vi "Parlog_creation.vi"(0 "DAC Range Setting":u8(knob)=3 scale=0.0..3.0, 1 "DAC and AD Settings":i32(slide)=3 scale=0.0..3.0, 2 "AD 7730 Bit Settings":i32(slide) scale=0.0..1.0, 3 "predicted time [ms] to finalize DAQ":dbl, 4 "Measured Time for DAQ [ms]":u32, 5 "start time":i64, 6 "single channel voltage factor":dbl=1.0, 7 "Single Channel Voltage Output AO":tag="Dev1/ao0", 8 "single channel number":i64=14, 10 "maximum voltage @ 10MW single channel":dbl=10.0 format="%#_13g", 14 "sample_rate":dbl, 15 "pulse_length":dbl, 16 "sample_period":dbl) -> (9 "chanDescs_defaultInd":T5(array[cluster])=[{"name"="HBCm_U30_01", "active"=1, "physicalQuantity"={"type"="A"}}, {"name"="HBCm_U30_02", "active"=1, "physicalQuantity"={"type"="A"}}, {"name"="HBCm_U30_03", "active"=1, "physicalQuantity"={"type"="A"}}, {"name"="HBCm_U30_04", "active"=1, "physicalQuantity"={"type"="A"}}, {"name"="HBCm_U30_05", "active"=1, "physicalQuantity"={"type"="A"}}, {"name"="HBCm_U30_06", "active"=1, "physicalQuantity"={"type"="A"}}, {"name"="HBCm_U30_07", "active"=1, "physicalQuantity"={"type"="A"}}, {"name"="HBCm_U30_08", "active"=1, "physicalQuantity"={"type"="A"}}, {"name"="HBCm_U30_09", "active"=1, "physicalQuantity"={"type"="A"}}, {"name"="HBCm_U30_10", "active"=1, "physicalQuantity"={"type"="A"}}, {"name"="HBCm_U30_11", "active"=1, "physicalQuantity"={"type"="A"}}, {"name"="HBCm_U30_12", "active"=1, "physicalQuantity"={"type"="A"}}, {"name"="HBCm_U30_13", "active"=1, "physicalQuantity"={"type"="A"}}, {"name"="HBCm_U30_14", "active"=1, "physicalQuantity"={"type"="A"}}, {"name"="HBCm_U30_15", "active"=1, "physicalQuantity"={"type"="A"}}, {"name"="HBCm_U30_16", "active"=1, "physicalQuantity"={"type"="A"}}, {"name"="HBCm_U30_17", "active"=1, "physicalQuantity"={"type"="A"}}, {"name"="HBCm_U30_18", "active"=1, "physicalQuantity"={"type"="A"}}, {"name"="HBCm_U30_19", "active"=1, "physicalQuantity"={"type"="A"}}, {"name"="HBCm_U30_20", "active"=1, "physicalQuantity"={"type"="A"}}, {"name"="HBCm_U30_21", "active"=1, "physicalQuantity"={"type"="A"}}, {"name"="HBCm_U30_22", "active"=1, "physicalQuantity"={"type"="A"}}, {"name"="HBCm_U30_23", "active"=1, "physicalQuantity"={"type"="A"}}, {"name"="HBCm_U30_24", "active"=1, "physicalQuantity"={"type"="A"}}, {"name"="HBCm_U30_25", "active"=1, "physicalQuantity"={"type"="A"}}, {"name"="HBCm_U30_26", "active"=1, "physicalQuantity"={"type"="A"}}, {"name"="HBCm_U30_27", "active"=1, "physicalQuantity"={"type"="A"}}, {"name"="HBCm_U30_28", "active"=1, "physicalQuantity"={"type"="A"}}, {"name"="HBCm_U30_29", "active"=1, "physicalQuantity"={"type"="A"}}, {"name"="HBCm_U30_30", "active"=1, "physicalQuantity"={"type"="A"}}, {"name"="HBCm_U30_31", "active"=1, "physicalQuantity"={"type"="A"}}, {"name"="HBCm_U30_32", "active"=1, "physicalQuantity"={"type"="A"}}, {"name"="VBCm_V21_01", "active"=1, "physicalQuantity"={"type"="A"}}, {"name"="VBCm_V21_02", "active"=1, "physicalQuantity"={"type"="A"}}, {"name"="VBCm_V21_03", "active"=1, "physicalQuantity"={"type"="A"}}, {"name"="VBCm_V21_04", "active"=1, "physicalQuantity"={"type"="A"}}, {"name"="VBCm_V21_05", "active"=1, "physicalQuantity"={"type"="A"}}, {"name"="VBCm_V21_06", "active"=1, "physicalQuantity"={"type"="A"}}, {"name"="VBCm_V21_07", "active"=1, "physicalQuantity"={"type"="A"}}, {"name"="VBCm_V21_08", "active"=1, "physicalQuantity"={"type"="A"}}, {"name"="VBCm_V21_09", "active"=1, "physicalQuantity"={"type"="A"}}, {"name"="VBCm_V21_10", "active"=1, "physicalQuantity"={"type"="A"}}, {"name"="VBCm_V21_11", "active"=1, "physicalQuantity"={"type"="A"}}, {"name"="VBCm_V21_12", "active"=1, "physicalQuantity"={"type"="A"}}, {"name"="VBCm_V21_13", "active"=1, "physicalQuantity"={"type"="A"}}, {"name"="VBCm_V21_14", "active"=1, "physicalQuantity"={"type"="A"}}, {"name"="VBCm_V21_15", "active"=1, "physicalQuantity"={"type"="A"}}, {"name"="VBCm_V21_16", "active"=1, "physicalQuantity"={"type"="A"}}, {"name"="VBCm_V21_17", "active"=1, "physicalQuantity"={"type"="A"}}, {"name"="VBCm_V21_18", "active"=1, "physicalQuantity"={"type"="A"}}, {"name"="VBCm_V21_19", "active"=1, "physicalQuantity"={"type"="A"}}, {"name"="VBCm_V21_20", "active"=1, "physicalQuantity"={"type"="A"}}, {"name"="VBCm_V21_21", "active"=1, "physicalQuantity"={"type"="A"}}, {"name"="VBCm_V21_22", "active"=1, "physicalQuantity"={"type"="A"}}, {"name"="VBCm_V21_23", "active"=1, "physicalQuantity"={"type"="A"}}, {"name"="VBCm_V21_24", "active"=1, "physicalQuantity"={"type"="A"}}, {"name"="VBCm_V21_25", "active"=1, "physicalQuantity"={"type"="A"}}, {"name"="VBCm_V21_26", "active"=1, "physicalQuantity"={"type"="A"}}, {"name"="VBCm_V21_27", "active"=1, "physicalQuantity"={"type"="A"}}, {"name"="VBCm_V21_28", "active"=1, "physicalQuantity"={"type"="A"}}, {"name"="VBCm_V21_29", "active"=1, "physicalQuantity"={"type"="A"}}, {"name"="VBCm_V21_30", "active"=1, "physicalQuantity"={"type"="A"}}, {"name"="VBCm_V21_31", "active"=1, "physicalQuantity"={"type"="A"}}, {"name"="VBCm_V21_32", "active"=1, "physicalQuantity"={"type"="A"}}, {"name"="VBCm_V21_33", "active"=1, "physicalQuantity"={"type"="A"}}, {"name"="VBCm_V21_34", "active"=1, "physicalQuantity"={"type"="A"}}, {"name"="VBCm_V21_35", "active"=1, "physicalQuantity"={"type"="A"}}, {"name"="VBCm_V21_36", "active"=1, "physicalQuantity"={"type"="A"}}, {"name"="VBCm_V21_37", "active"=1, "physicalQuantity"={"type"="A"}}, {"name"="VBCm_V21_38", "active"=1, "physicalQuantity"={"type"="A"}}, {"name"="VBCm_V21_39", "active"=1, "physicalQuantity"={"type"="A"}}, {"name"="VBCm_V21_40", "active"=1, "physicalQuantity"={"type"="A"}}, {"name"="VBCs_V21_01", "active"=1, "physicalQuantity"={"type"="A"}}, {"name"="VBCs_V21_02", "active"=1, "physicalQuantity"={"type"="A"}}, {"name"="VBCs_V21_03", "active"=1, "physicalQuantity"={"type"="A"}}, {"name"="VBCs_V21_04", "active"=1, "physicalQuantity"={"type"="A"}}, {"name"="VBCs_V21_05", "active"=1, "physicalQuantity"={"type"="A"}}, {"name"="VBCs_V21_06", "active"=1, "physicalQuantity"={"type"="A"}}, {"name"="VBCs_V21_07", "active"=1, "physicalQuantity"={"type"="A"}}, {"name"="VBCs_V21_08", "active"=1, "physicalQuantity"={"type"="A"}}, {"name"="HBCs_U30_01", "active"=1, "physicalQuantity"={"type"="A"}}, {"name"="HBCs_U30_02", "active"=1, "physicalQuantity"={"type"="A"}}, {"name"="HBCs_U30_03", "active"=1, "physicalQuantity"={"type"="A"}}, {"name"="HBCs_U30_04", "active"=1, "physicalQuantity"={"type"="A"}}, {"name"="HBCs_U30_05", "active"=1, "physicalQuantity"={"type"="A"}}, {"name"="HBCs_U30_06", "active"=1, "physicalQuantity"={"type"="A"}}, {"name"="HBCs_U30_07", "active"=1, "physicalQuantity"={"type"="A"}}, {"name"="HBCs_U30_08", "active"=1, "physicalQuantity"={"type"="A"}}, {"name"="HBCs_U30_09", "active"=1, "physicalQuantity"={"type"="A"}}, {"name"="HBCs_U30_10", "active"=1, "physicalQuantity"={"type"="A"}}, {"name"="HBCs_U30_11", "active"=1, "physicalQuantity"={"type"="A"}}, {"name"="HBCs_U30_12", "active"=1, "physicalQuantity"={"type"="A"}}, {"name"="HBCs_U30_13", "active"=1, "physicalQuantity"={"type"="A"}}, {"name"="HBCs_U30_14", "active"=1, "physicalQuantity"={"type"="A"}}, {"name"="HBCs_U30_15", "active"=1, "physicalQuantity"={"type"="A"}}, {"name"="HBCs_U30_16", "active"=1, "physicalQuantity"={"type"="A"}}, {"name"="Test96", "active"=1, "physicalQuantity"={"type"="A"}}, {"name"="Test97", "active"=0, "physicalQuantity"={"type"=""}}], 11 "chanDescs_ArrayOfArray":T6(array[cluster])=[{"chanDescs"=[{"name"="E_Chan_1", "active"=1}, {"name"="E_Chan_2", "active"=1}, {"name"="E_Chan_3", "active"=1}, {"name"="E_Chan_4", "active"=1}, {"name"="E_Chan_5", "active"=1}, {"name"="E_Chan_6", "active"=1}, {"name"="E_Chan_7", "active"=1}, {"name"="E_Chan_8", "active"=1}, {"name"="E_Chan_9", "active"=1}, {"name"="E_Chan_10", "active"=1}, {"name"="E_Chan_11", "active"=1}, {"name"="E_Chan_12", "active"=1}, {"name"="E_Chan_13", "active"=1}, {"name"="E_Chan_14", "active"=1}, {"name"="E_Chan_15", "active"=1}, {"name"="E_Chan_16", "active"=1}, {"name"="E_Chan_17", "active"=1}, {"name"="E_Chan_18", "active"=1}, {"name"="E_Chan_19", "active"=1}, {"name"="E_Chan_20", "active"=1}, {"name"="E_Chan_21", "active"=1}, {"name"="E_Chan_22", "active"=1}, {"name"="E_Chan_23", "active"=1}, {"name"="E_Chan_24", "active"=1}, {"name"="E_Chan_25", "active"=1}, {"name"="E_Chan_26", "active"=1}, {"name"="E_Chan_27", "active"=1}, {"name"="E_Chan_28", "active"=1}, {"name"="E_Chan_29", "active"=1}, {"name"="E_Chan_30", "active"=1}, {"name"="E_Chan_31", "active"=1}, {"name"="E_Chan_32", "active"=1}, {"name"="E_Chan_33", "active"=1}, {"name"="E_Chan_34", "active"=1}, {"name"="E_Chan_35", "active"=1}, {"name"="E_Chan_36", "active"=1}, {"name"="E_Chan_37", "active"=1}, {"name"="E_Chan_38", "active"=1}, {"name"="E_Chan_39", "active"=1}, {"name"="E_Chan_40", "active"=1}, {"name"="E_Chan_41", "active"=1}, {"name"="E_Chan_42", "active"=1}, {"name"="E_Chan_43", "active"=1}, {"name"="E_Chan_44", "active"=1}, {"name"="E_Chan_45", "active"=1}, {"name"="E_Chan_46", "active"=1}, {"name"="E_Chan_47", "active"=1}, {"name"="E_Chan_48", "active"=1}, {"name"="E_Chan_49", "active"=1}, {"name"="E_Chan_50", "active"=1}, {"name"="E_Chan_51", "active"=1}, {"name"="E_Chan_52", "active"=1}, {"name"="E_Chan_53", "active"=1}, {"name"="E_Chan_54", "active"=1}, {"name"="E_Chan_55", "active"=1}, {"name"="E_Chan_56", "active"=1}, {"name"="E_Chan_57", "active"=1}, {"name"="E_Chan_58", "active"=1}, {"name"="E_Chan_59", "active"=1}, {"name"="E_Chan_60", "active"=1}, {"name"="E_Chan_61", "active"=1}, {"name"="E_Chan_62", "active"=1}, {"name"="E_Chan_63", "active"=1}, {"name"="E_Chan_64", "active"=1}, {"name"="E_Chan_65", "active"=1}, {"name"="E_Chan_66", "active"=1}, {"name"="E_Chan_67", "active"=1}, {"name"="E_Chan_68", "active"=1}, {"name"="E_Chan_69", "active"=1}, {"name"="E_Chan_70", "active"=1}, {"name"="E_Chan_71", "active"=1}, {"name"="E_Chan_72", "active"=1}, {"name"="E_Chan_73", "active"=1}, {"name"="E_Chan_74", "active"=1}, {"name"="E_Chan_75", "active"=1}, {"name"="E_Chan_76", "active"=1}, {"name"="E_Chan_77", "active"=1}, {"name"="E_Chan_78", "active"=1}, {"name"="E_Chan_79", "active"=1}, {"name"="E_Chan_80", "active"=1}, {"name"="E_Chan_81", "active"=1}, {"name"="E_Chan_82", "active"=1}, {"name"="E_Chan_83", "active"=1}, {"name"="E_Chan_84", "active"=1}, {"name"="E_Chan_85", "active"=1}, {"name"="E_Chan_86", "active"=1}, {"name"="E_Chan_87", "active"=1}, {"name"="E_Chan_88", "active"=1}, {"name"="E_Chan_89", "active"=1}, {"name"="E_Chan_90", "active"=1}, {"name"="E_Chan_91", "active"=1}, {"name"="E_Chan_92", "active"=1}, {"name"="E_Chan_93", "active"=1}, {"name"="E_Chan_94", "active"=1}, {"name"="E_Chan_95", "active"=1}, {"name"="E_Chan_96", "active"=1}, {"name"="E_Chan_97", "active"=1}, {"name"="E_Chan_98", "active"=1}, {"name"="E_Chan_99", "active"=1}, {"name"="E_Chan_100", "active"=1}, {"name"="E_Chan_101", "active"=1}, {"name"="E_Chan_102", "active"=1}, {"name"="E_Chan_103", "active"=1}, {"name"="E_Chan_104", "active"=1}, {"name"="E_Chan_105", "active"=1}, {"name"="E_Chan_106", "active"=1}, {"name"="E_Chan_107", "active"=1}, {"name"="E_Chan_108", "active"=1}, {"name"="E_Chan_109", "active"=1}, {"name"="E_Chan_110", "active"=1}, {"name"="E_Chan_111", "active"=1}, {"name"="E_Chan_112", "active"=1}, {"name"="E_Chan_113", "active"=1}, {"name"="E_Chan_114", "active"=1}, {"name"="E_Chan_115", "active"=1}, {"name"="E_Chan_116", "active"=1}, {"name"="E_Chan_117", "active"=1}, {"name"="E_Chan_118", "active"=1}, {"name"="E_Chan_119", "active"=1}, {"name"="E_Chan_120", "active"=1}, {"name"="E_Chan_121", "active"=1}, {"name"="E_Chan_122", "active"=1}, {"name"="E_Chan_123", "active"=1}, {"name"="E_Chan_124", "active"=1}, {"name"="E_Chan_125", "active"=1}, {"name"="E_Chan_126", "active"=1}, {"name"="E_Chan_127", "active"=1}, {"name"="E_Chan_128", "active"=1}]}], 12 "cluster":T1, 13 "reduced cluster array":T3(array[cluster]), 17 "reduced cluster":T4, 18 "chanDescsInd":T5(array[cluster])=[{"name"="HBCm_U30_01", "active"=1, "physicalQuantity"={"type"="A"}}, {"name"="HBCm_U30_02", "active"=1, "physicalQuantity"={"type"="A"}}, {"name"="HBCm_U30_03", "active"=1, "physicalQuantity"={"type"="A"}}, {"name"="HBCm_U30_04", "active"=1, "physicalQuantity"={"type"="A"}}, {"name"="HBCm_U30_05", "active"=1, "physicalQuantity"={"type"="A"}}, {"name"="HBCm_U30_06", "active"=1, "physicalQuantity"={"type"="A"}}, {"name"="HBCm_U30_07", "active"=1, "physicalQuantity"={"type"="A"}}, {"name"="HBCm_U30_08", "active"=1, "physicalQuantity"={"type"="A"}}, {"name"="HBCm_U30_09", "active"=1, "physicalQuantity"={"type"="A"}}, {"name"="HBCm_U30_10", "active"=1, "physicalQuantity"={"type"="A"}}, {"name"="HBCm_U30_11", "active"=1, "physicalQuantity"={"type"="A"}}, {"name"="HBCm_U30_12", "active"=1, "physicalQuantity"={"type"="A"}}, {"name"="HBCm_U30_013", "active"=1, "physicalQuantity"={"type"="A"}}, {"name"="HBCm_U30_14", "active"=1, "physicalQuantity"={"type"="A"}}, {"name"="HBCm_U30_15", "active"=1, "physicalQuantity"={"type"="A"}}, {"name"="HBCm_U30_16", "active"=1, "physicalQuantity"={"type"="A"}}, {"name"="HBCm_U30_17", "active"=1, "physicalQuantity"={"type"="A"}}, {"name"="HBCm_U30_18", "active"=1, "physicalQuantity"={"type"="A"}}, {"name"="HBCm_U30_19", "active"=1, "physicalQuantity"={"type"="A"}}, {"name"="HBCm_U30_20", "active"=1, "physicalQuantity"={"type"="A"}}, {"name"="HBCm_U30_21", "active"=1, "physicalQuantity"={"type"="A"}}, {"name"="HBCm_U30_22", "active"=1, "physicalQuantity"={"type"="A"}}, {"name"="HBCm_U30_23", "active"=1, "physicalQuantity"={"type"="A"}}, {"name"="HBCm_U30_24", "active"=1, "physicalQuantity"={"type"="A"}}, {"name"="HBCm_U30_25", "active"=1, "physicalQuantity"={"type"="A"}}, {"name"="HBCm_U30_26", "active"=1, "physicalQuantity"={"type"="A"}}, {"name"="HBCm_U30_27", "active"=1, "physicalQuantity"={"type"="A"}}, {"name"="HBCm_U30_28", "active"=1, "physicalQuantity"={"type"="A"}}, {"name"="HBCm_U30_29", "active"=1, "physicalQuantity"={"type"="A"}}, {"name"="HBCm_U30_30", "active"=1, "physicalQuantity"={"type"="A"}}, {"name"="HBCm_U30_31", "active"=1, "physicalQuantity"={"type"="A"}}, {"name"="HBCm_U30_32", "active"=1, "physicalQuantity"={"type"="A"}}, {"name"="VBCm_V21_01", "active"=1, "physicalQuantity"={"type"="A"}}, {"name"="VBCm_V21_02", "active"=1, "physicalQuantity"={"type"="A"}}, {"name"="VBCm_V21_03", "active"=1, "physicalQuantity"={"type"="A"}}, {"name"="VBCm_V21_04", "active"=1, "physicalQuantity"={"type"="A"}}, {"name"="VBCm_V21_05", "active"=1, "physicalQuantity"={"type"="A"}}, {"name"="VBCm_V21_06", "active"=1, "physicalQuantity"={"type"="A"}}, {"name"="VBCm_V21_07", "active"=1, "physicalQuantity"={"type"="A"}}, {"name"="VBCm_V21_08", "active"=1, "physicalQuantity"={"type"="A"}}, {"name"="VBCm_V21_09", "active"=1, "physicalQuantity"={"type"="A"}}, {"name"="VBCm_V21_10", "active"=1, "physicalQuantity"={"type"="A"}}, {"name"="VBCm_V21_11", "active"=1, "physicalQuantity"={"type"="A"}}, {"name"="VBCm_V21_12", "active"=1, "physicalQuantity"={"type"="A"}}, {"name"="VBCm_V21_13", "active"=1, "physicalQuantity"={"type"="A"}}, {"name"="VBCm_V21_14", "active"=1, "physicalQuantity"={"type"="A"}}, {"name"="VBCm_V21_15", "active"=1, "physicalQuantity"={"type"="A"}}, {"name"="VBCm_V21_16", "active"=1, "physicalQuantity"={"type"="A"}}, {"name"="VBCm_V21_17", "active"=1, "physicalQuantity"={"type"="A"}}, {"name"="VBCm_V21_18", "active"=1, "physicalQuantity"={"type"="A"}}, {"name"="VBCm_V21_19", "active"=1, "physicalQuantity"={"type"="A"}}, {"name"="VBCm_V21_20", "active"=1, "physicalQuantity"={"type"="A"}}, {"name"="VBCm_V21_21", "active"=1, "physicalQuantity"={"type"="A"}}, {"name"="VBCm_V21_22", "active"=1, "physicalQuantity"={"type"="A"}}, {"name"="VBCm_V21_23", "active"=1, "physicalQuantity"={"type"="A"}}, {"name"="VBCm_V21_24", "active"=1, "physicalQuantity"={"type"="A"}}, {"name"="VBCm_V21_25", "active"=1, "physicalQuantity"={"type"="A"}}, {"name"="VBCm_V21_26", "active"=1, "physicalQuantity"={"type"="A"}}, {"name"="VBCm_V21_27", "active"=1, "physicalQuantity"={"type"="A"}}, {"name"="VBCm_V21_28", "active"=1, "physicalQuantity"={"type"="A"}}, {"name"="VBCm_V21_29", "active"=1, "physicalQuantity"={"type"="A"}}, {"name"="VBCm_V21_30", "active"=1, "physicalQuantity"={"type"="A"}}, {"name"="VBCm_V21_31", "active"=1, "physicalQuantity"={"type"="A"}}, {"name"="VBCm_V21_32", "active"=1, "physicalQuantity"={"type"="A"}}, {"name"="VBCm_V21_33", "active"=1, "physicalQuantity"={"type"="A"}}, {"name"="VBCm_V21_34", "active"=1, "physicalQuantity"={"type"="A"}}, {"name"="VBCm_V21_35", "active"=1, "physicalQuantity"={"type"="A"}}, {"name"="VBCm_V21_36", "active"=1, "physicalQuantity"={"type"="A"}}, {"name"="VBCm_V21_37", "active"=1, "physicalQuantity"={"type"="A"}}, {"name"="VBCm_V21_38", "active"=1, "physicalQuantity"={"type"="A"}}, {"name"="VBCm_V21_39", "active"=1, "physicalQuantity"={"type"="A"}}, {"name"="VBCm_V21_40", "active"=1, "physicalQuantity"={"type"="A"}}, {"name"="VBCs_V21_01", "active"=1, "physicalQuantity"={"type"="A"}}, {"name"="VBCs_V21_02", "active"=1, "physicalQuantity"={"type"="A"}}, {"name"="VBCs_V21_03", "active"=1, "physicalQuantity"={"type"="A"}}, {"name"="VBCs_V21_04", "active"=1, "physicalQuantity"={"type"="A"}}, {"name"="VBCs_V21_05", "active"=1, "physicalQuantity"={"type"="A"}}, {"name"="VBCs_V21_06", "active"=1, "physicalQuantity"={"type"="A"}}, {"name"="VBCs_V21_07", "active"=1, "physicalQuantity"={"type"="A"}}, {"name"="VBCs_V21_08", "active"=1, "physicalQuantity"={"type"="A"}}, {"name"="HBCs_U30_01", "active"=1, "physicalQuantity"={"type"="A"}}, {"name"="HBCs_U30_02", "active"=1, "physicalQuantity"={"type"="A"}}, {"name"="HBCs_U30_03", "active"=1, "physicalQuantity"={"type"="A"}}, {"name"="HBCs_U30_04", "active"=1, "physicalQuantity"={"type"="A"}}, {"name"="HBCs_U30_05", "active"=1, "physicalQuantity"={"type"="A"}}, {"name"="HBCs_U30_06", "active"=1, "physicalQuantity"={"type"="A"}}, {"name"="HBCs_U30_07", "active"=1, "physicalQuantity"={"type"="A"}}, {"name"="HBCs_U30_08", "active"=1, "physicalQuantity"={"type"="A"}}, {"name"="HBCs_U30_09", "active"=1, "physicalQuantity"={"type"="A"}}, {"name"="HBCs_U30_10", "active"=1, "physicalQuantity"={"type"="A"}}, {"name"="HBCs_U30_11", "active"=1, "physicalQuantity"={"type"="A"}}, {"name"="HBCs_U30_12", "active"=1, "physicalQuantity"={"type"="A"}}, {"name"="HBCs_U30_13", "active"=1, "physicalQuantity"={"type"="A"}}, {"name"="HBCs_U30_14", "active"=1, "physicalQuantity"={"type"="A"}}, {"name"="HBCs_U30_15", "active"=1, "physicalQuantity"={"type"="A"}}, {"name"="HBCs_U30_16", "active"=1, "physicalQuantity"={"type"="A"}}], 19 "cluster array":T2(array[cluster]))   [LabVIEW 2014]
panel:
  out "cluster json":string
  out "cluster array json":string
  out "chanDescs 2":cluster{"name":string, "active":i32}[](array[cluster])=[{"name"="E_Chan_1", "active"=1}, {"name"="E_Chan_2", "active"=1}, {"name"="E_Chan_3", "active"=1}, {"name"="E_Chan_4", "active"=1}, {"name"="E_Chan_5", "active"=1}, {"name"="E_Chan_6", "active"=1}, {"name"="E_Chan_7", "active"=1}, {"name"="E_Chan_8", "active"=1}, {"name"="E_Chan_9", "active"=1}, {"name"="E_Chan_10", "active"=1}, {"name"="E_Chan_11", "active"=1}, {"name"="E_Chan_12", "active"=1}, {"name"="E_Chan_13", "active"=1}, {"name"="E_Chan_14", "active"=1}, {"name"="E_Chan_15", "active"=1}, {"name"="E_Chan_16", "active"=1}, {"name"="E_Chan_17", "active"=1}, {"name"="E_Chan_18", "active"=1}, {"name"="E_Chan_19", "active"=1}, {"name"="E_Chan_20", "active"=1}, {"name"="E_Chan_21", "active"=1}, {"name"="E_Chan_22", "active"=1}, {"name"="E_Chan_23", "active"=1}, {"name"="E_Chan_24", "active"=1}, {"name"="E_Chan_25", "active"=1}, {"name"="E_Chan_26", "active"=1}, {"name"="E_Chan_27", "active"=1}, {"name"="E_Chan_28", "active"=1}, {"name"="E_Chan_29", "active"=1}, {"name"="E_Chan_30", "active"=1}, {"name"="E_Chan_31", "active"=1}, {"name"="E_Chan_32", "active"=1}, {"name"="E_Chan_33", "active"=1}, {"name"="E_Chan_34", "active"=1}, {"name"="E_Chan_35", "active"=1}, {"name"="E_Chan_36", "active"=1}, {"name"="E_Chan_37", "active"=1}, {"name"="E_Chan_38", "active"=1}, {"name"="E_Chan_39", "active"=1}, {"name"="E_Chan_40", "active"=1}, {"name"="E_Chan_41", "active"=1}, {"name"="E_Chan_42", "active"=1}, {"name"="E_Chan_43", "active"=1}, {"name"="E_Chan_44", "active"=1}, {"name"="E_Chan_45", "active"=1}, {"name"="E_Chan_46", "active"=1}, {"name"="E_Chan_47", "active"=1}, {"name"="E_Chan_48", "active"=1}, {"name"="E_Chan_49", "active"=1}, {"name"="E_Chan_50", "active"=1}, {"name"="E_Chan_51", "active"=1}, {"name"="E_Chan_52", "active"=1}, {"name"="E_Chan_53", "active"=1}, {"name"="E_Chan_54", "active"=1}, {"name"="E_Chan_55", "active"=1}, {"name"="E_Chan_56", "active"=1}, {"name"="E_Chan_57", "active"=1}, {"name"="E_Chan_58", "active"=1}, {"name"="E_Chan_59", "active"=1}, {"name"="E_Chan_60", "active"=1}, {"name"="E_Chan_61", "active"=1}, {"name"="E_Chan_62", "active"=1}, {"name"="E_Chan_63", "active"=1}, {"name"="E_Chan_64", "active"=1}, {"name"="E_Chan_65", "active"=1}, {"name"="E_Chan_66", "active"=1}, {"name"="E_Chan_67", "active"=1}, {"name"="E_Chan_68", "active"=1}, {"name"="E_Chan_69", "active"=1}, {"name"="E_Chan_70", "active"=1}, {"name"="E_Chan_71", "active"=1}, {"name"="E_Chan_72", "active"=1}, {"name"="E_Chan_73", "active"=1}, {"name"="E_Chan_74", "active"=1}, {"name"="E_Chan_75", "active"=1}, {"name"="E_Chan_76", "active"=1}, {"name"="E_Chan_77", "active"=1}, {"name"="E_Chan_78", "active"=1}, {"name"="E_Chan_79", "active"=1}, {"name"="E_Chan_80", "active"=1}, {"name"="E_Chan_81", "active"=1}, {"name"="E_Chan_82", "active"=1}, {"name"="E_Chan_83", "active"=1}, {"name"="E_Chan_84", "active"=1}, {"name"="E_Chan_85", "active"=1}, {"name"="E_Chan_86", "active"=1}, {"name"="E_Chan_87", "active"=1}, {"name"="E_Chan_88", "active"=1}, {"name"="E_Chan_89", "active"=1}, {"name"="E_Chan_90", "active"=1}, {"name"="E_Chan_91", "active"=1}, {"name"="E_Chan_92", "active"=1}, {"name"="E_Chan_93", "active"=1}, {"name"="E_Chan_94", "active"=1}, {"name"="E_Chan_95", "active"=1}, {"name"="E_Chan_96", "active"=1}, {"name"="E_Chan_97", "active"=1}, {"name"="E_Chan_98", "active"=1}, {"name"="E_Chan_99", "active"=1}, {"name"="E_Chan_100", "active"=1}, {"name"="E_Chan_101", "active"=1}, {"name"="E_Chan_102", "active"=1}, {"name"="E_Chan_103", "active"=1}, {"name"="E_Chan_104", "active"=1}, {"name"="E_Chan_105", "active"=1}, {"name"="E_Chan_106", "active"=1}, {"name"="E_Chan_107", "active"=1}, {"name"="E_Chan_108", "active"=1}, {"name"="E_Chan_109", "active"=1}, {"name"="E_Chan_110", "active"=1}, {"name"="E_Chan_111", "active"=1}, {"name"="E_Chan_112", "active"=1}, {"name"="E_Chan_113", "active"=1}, {"name"="E_Chan_114", "active"=1}, {"name"="E_Chan_115", "active"=1}, {"name"="E_Chan_116", "active"=1}, {"name"="E_Chan_117", "active"=1}, {"name"="E_Chan_118", "active"=1}, {"name"="E_Chan_119", "active"=1}, {"name"="E_Chan_120", "active"=1}, {"name"="E_Chan_121", "active"=1}, {"name"="E_Chan_122", "active"=1}, {"name"="E_Chan_123", "active"=1}, {"name"="E_Chan_124", "active"=1}, {"name"="E_Chan_125", "active"=1}, {"name"="E_Chan_126", "active"=1}, {"name"="E_Chan_127", "active"=1}, {"name"="E_Chan_128", "active"=1}]
  in  "chanDescs":T5(array[cluster])=[{"name"="HBCm_U30_01", "active"=1, "physicalQuantity"={"type"="A"}}, {"name"="HBCm_U30_02", "active"=1, "physicalQuantity"={"type"="A"}}, {"name"="HBCm_U30_03", "active"=1, "physicalQuantity"={"type"="A"}}, {"name"="HBCm_U30_04", "active"=1, "physicalQuantity"={"type"="A"}}, {"name"="HBCm_U30_05", "active"=1, "physicalQuantity"={"type"="A"}}, {"name"="HBCm_U30_06", "active"=1, "physicalQuantity"={"type"="A"}}, {"name"="HBCm_U30_07", "active"=1, "physicalQuantity"={"type"="A"}}, {"name"="HBCm_U30_08", "active"=1, "physicalQuantity"={"type"="A"}}, {"name"="HBCm_U30_09", "active"=1, "physicalQuantity"={"type"="A"}}, {"name"="HBCm_U30_10", "active"=1, "physicalQuantity"={"type"="A"}}, {"name"="HBCm_U30_11", "active"=1, "physicalQuantity"={"type"="A"}}, {"name"="HBCm_U30_12", "active"=1, "physicalQuantity"={"type"="A"}}, {"name"="HBCm_U30_013", "active"=1, "physicalQuantity"={"type"="A"}}, {"name"="HBCm_U30_14", "active"=1, "physicalQuantity"={"type"="A"}}, {"name"="HBCm_U30_15", "active"=1, "physicalQuantity"={"type"="A"}}, {"name"="HBCm_U30_16", "active"=1, "physicalQuantity"={"type"="A"}}, {"name"="HBCm_U30_17", "active"=1, "physicalQuantity"={"type"="A"}}, {"name"="HBCm_U30_18", "active"=1, "physicalQuantity"={"type"="A"}}, {"name"="HBCm_U30_19", "active"=1, "physicalQuantity"={"type"="A"}}, {"name"="HBCm_U30_20", "active"=1, "physicalQuantity"={"type"="A"}}, {"name"="HBCm_U30_21", "active"=1, "physicalQuantity"={"type"="A"}}, {"name"="HBCm_U30_22", "active"=1, "physicalQuantity"={"type"="A"}}, {"name"="HBCm_U30_23", "active"=1, "physicalQuantity"={"type"="A"}}, {"name"="HBCm_U30_24", "active"=1, "physicalQuantity"={"type"="A"}}, {"name"="HBCm_U30_25", "active"=1, "physicalQuantity"={"type"="A"}}, {"name"="HBCm_U30_26", "active"=1, "physicalQuantity"={"type"="A"}}, {"name"="HBCm_U30_27", "active"=1, "physicalQuantity"={"type"="A"}}, {"name"="HBCm_U30_28", "active"=1, "physicalQuantity"={"type"="A"}}, {"name"="HBCm_U30_29", "active"=1, "physicalQuantity"={"type"="A"}}, {"name"="HBCm_U30_30", "active"=1, "physicalQuantity"={"type"="A"}}, {"name"="HBCm_U30_31", "active"=1, "physicalQuantity"={"type"="A"}}, {"name"="HBCm_U30_32", "active"=1, "physicalQuantity"={"type"="A"}}, {"name"="VBCm_V21_01", "active"=1, "physicalQuantity"={"type"="A"}}, {"name"="VBCm_V21_02", "active"=1, "physicalQuantity"={"type"="A"}}, {"name"="VBCm_V21_03", "active"=1, "physicalQuantity"={"type"="A"}}, {"name"="VBCm_V21_04", "active"=1, "physicalQuantity"={"type"="A"}}, {"name"="VBCm_V21_05", "active"=1, "physicalQuantity"={"type"="A"}}, {"name"="VBCm_V21_06", "active"=1, "physicalQuantity"={"type"="A"}}, {"name"="VBCm_V21_07", "active"=1, "physicalQuantity"={"type"="A"}}, {"name"="VBCm_V21_08", "active"=1, "physicalQuantity"={"type"="A"}}, {"name"="VBCm_V21_09", "active"=1, "physicalQuantity"={"type"="A"}}, {"name"="VBCm_V21_10", "active"=1, "physicalQuantity"={"type"="A"}}, {"name"="VBCm_V21_11", "active"=1, "physicalQuantity"={"type"="A"}}, {"name"="VBCm_V21_12", "active"=1, "physicalQuantity"={"type"="A"}}, {"name"="VBCm_V21_13", "active"=1, "physicalQuantity"={"type"="A"}}, {"name"="VBCm_V21_14", "active"=1, "physicalQuantity"={"type"="A"}}, {"name"="VBCm_V21_15", "active"=1, "physicalQuantity"={"type"="A"}}, {"name"="VBCm_V21_16", "active"=1, "physicalQuantity"={"type"="A"}}, {"name"="VBCm_V21_17", "active"=1, "physicalQuantity"={"type"="A"}}, {"name"="VBCm_V21_18", "active"=1, "physicalQuantity"={"type"="A"}}, {"name"="VBCm_V21_19", "active"=1, "physicalQuantity"={"type"="A"}}, {"name"="VBCm_V21_20", "active"=1, "physicalQuantity"={"type"="A"}}, {"name"="VBCm_V21_21", "active"=1, "physicalQuantity"={"type"="A"}}, {"name"="VBCm_V21_22", "active"=1, "physicalQuantity"={"type"="A"}}, {"name"="VBCm_V21_23", "active"=1, "physicalQuantity"={"type"="A"}}, {"name"="VBCm_V21_24", "active"=1, "physicalQuantity"={"type"="A"}}, {"name"="VBCm_V21_25", "active"=1, "physicalQuantity"={"type"="A"}}, {"name"="VBCm_V21_26", "active"=1, "physicalQuantity"={"type"="A"}}, {"name"="VBCm_V21_27", "active"=1, "physicalQuantity"={"type"="A"}}, {"name"="VBCm_V21_28", "active"=1, "physicalQuantity"={"type"="A"}}, {"name"="VBCm_V21_29", "active"=1, "physicalQuantity"={"type"="A"}}, {"name"="VBCm_V21_30", "active"=1, "physicalQuantity"={"type"="A"}}, {"name"="VBCm_V21_31", "active"=1, "physicalQuantity"={"type"="A"}}, {"name"="VBCm_V21_32", "active"=1, "physicalQuantity"={"type"="A"}}, {"name"="VBCm_V21_33", "active"=1, "physicalQuantity"={"type"="A"}}, {"name"="VBCm_V21_34", "active"=1, "physicalQuantity"={"type"="A"}}, {"name"="VBCm_V21_35", "active"=1, "physicalQuantity"={"type"="A"}}, {"name"="VBCm_V21_36", "active"=1, "physicalQuantity"={"type"="A"}}, {"name"="VBCm_V21_37", "active"=1, "physicalQuantity"={"type"="A"}}, {"name"="VBCm_V21_38", "active"=1, "physicalQuantity"={"type"="A"}}, {"name"="VBCm_V21_39", "active"=1, "physicalQuantity"={"type"="A"}}, {"name"="VBCm_V21_40", "active"=1, "physicalQuantity"={"type"="A"}}, {"name"="VBCs_V21_01", "active"=1, "physicalQuantity"={"type"="A"}}, {"name"="VBCs_V21_02", "active"=1, "physicalQuantity"={"type"="A"}}, {"name"="VBCs_V21_03", "active"=1, "physicalQuantity"={"type"="A"}}, {"name"="VBCs_V21_04", "active"=1, "physicalQuantity"={"type"="A"}}, {"name"="VBCs_V21_05", "active"=1, "physicalQuantity"={"type"="A"}}, {"name"="VBCs_V21_06", "active"=1, "physicalQuantity"={"type"="A"}}, {"name"="VBCs_V21_07", "active"=1, "physicalQuantity"={"type"="A"}}, {"name"="VBCs_V21_08", "active"=1, "physicalQuantity"={"type"="A"}}, {"name"="HBCs_U30_01", "active"=1, "physicalQuantity"={"type"="A"}}, {"name"="HBCs_U30_02", "active"=1, "physicalQuantity"={"type"="A"}}, {"name"="HBCs_U30_03", "active"=1, "physicalQuantity"={"type"="A"}}, {"name"="HBCs_U30_04", "active"=1, "physicalQuantity"={"type"="A"}}, {"name"="HBCs_U30_05", "active"=1, "physicalQuantity"={"type"="A"}}, {"name"="HBCs_U30_06", "active"=1, "physicalQuantity"={"type"="A"}}, {"name"="HBCs_U30_07", "active"=1, "physicalQuantity"={"type"="A"}}, {"name"="HBCs_U30_08", "active"=1, "physicalQuantity"={"type"="A"}}, {"name"="HBCs_U30_09", "active"=1, "physicalQuantity"={"type"="A"}}, {"name"="HBCs_U30_10", "active"=1, "physicalQuantity"={"type"="A"}}, {"name"="HBCs_U30_11", "active"=1, "physicalQuantity"={"type"="A"}}, {"name"="HBCs_U30_12", "active"=1, "physicalQuantity"={"type"="A"}}, {"name"="HBCs_U30_13", "active"=1, "physicalQuantity"={"type"="A"}}, {"name"="HBCs_U30_14", "active"=1, "physicalQuantity"={"type"="A"}}, {"name"="HBCs_U30_15", "active"=1, "physicalQuantity"={"type"="A"}}, {"name"="HBCs_U30_16", "active"=1, "physicalQuantity"={"type"="A"}}]
  in  "Pre-start time (ms) of DAQ Typically set to 1000 ms":i32=5000
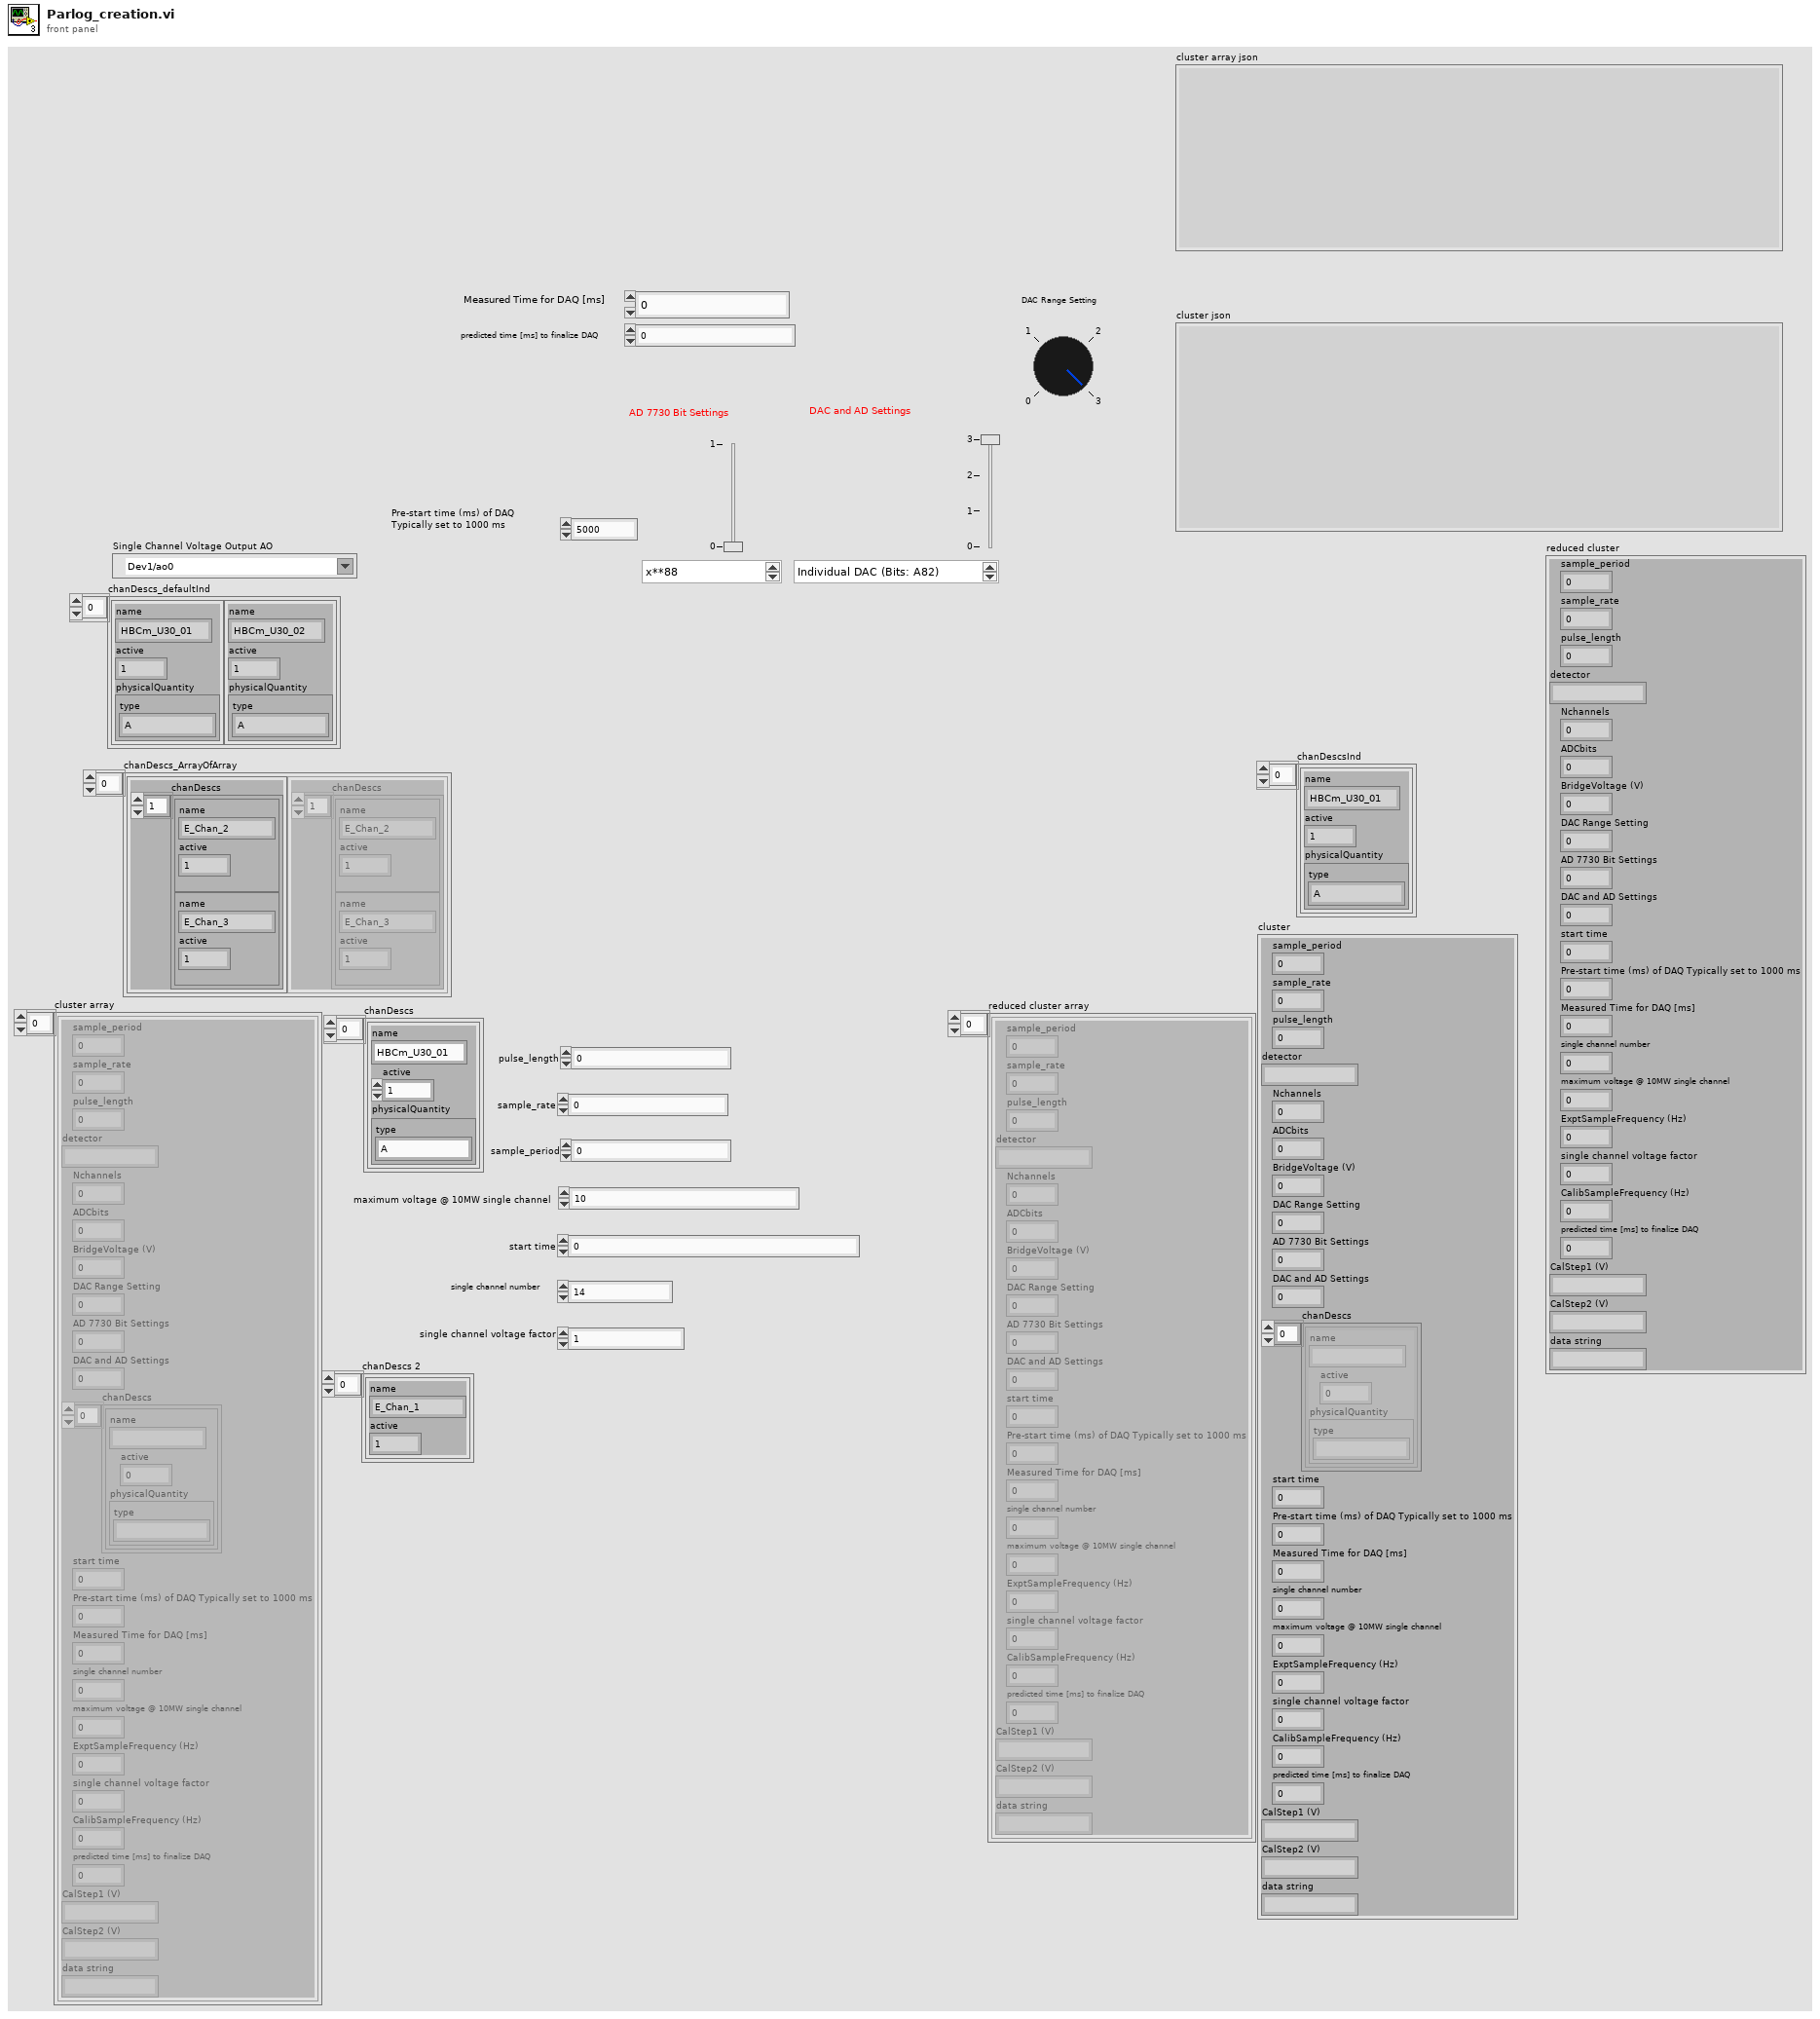
[diagram p1: front panel]
types:
  T1 = cluster{"sample_period":dbl, "sample_rate":dbl, "pulse_length":dbl, "detector":string, "Nchannels":i16, "ADCbits":i16, "BridgeVoltage (V)":sgl, "DAC Range Setting":u8, "AD 7730 Bit Settings":i32, "DAC and AD Settings":i32, "chanDescs":cluster{"name":string, "active":i32, "physicalQuantity":cluster{"type":string}}[], "start time":i64, "Pre-start time (ms) of DAQ Typically set to 1000 ms":i32, "Measured Time for DAQ [ms] ":u32, "single channel number":i64, "maximum voltage @ 10MW single channel":dbl, "ExptSampleFrequency (Hz)":sgl, "single channel voltage factor":dbl, "CalibSampleFrequency (Hz)":sgl, "predicted time [ms] to finalize DAQ":dbl, "CalStep1 (V)":string, "CalStep2 (V)":string, "data string":string}
  T2 = cluster{"sample_period":dbl, "sample_rate":dbl, "pulse_length":dbl, "detector":string, "Nchannels":i16, "ADCbits":i16, "BridgeVoltage (V)":sgl, "DAC Range Setting":u8, "AD 7730 Bit Settings":i32, "DAC and AD Settings":i32, "chanDescs":cluster{"name":string, "active":i32, "physicalQuantity":cluster{"type":string}}[], "start time":i64, "Pre-start time (ms) of DAQ Typically set to 1000 ms":i32, "Measured Time for DAQ [ms] ":u32, "single channel number":i64, "maximum voltage @ 10MW single channel":dbl, "ExptSampleFrequency (Hz)":sgl, "single channel voltage factor":dbl, "CalibSampleFrequency (Hz)":sgl, "predicted time [ms] to finalize DAQ":dbl, "CalStep1 (V)":string, "CalStep2 (V)":string, "data string":string}[]
  T3 = cluster{"sample_period":dbl, "sample_rate":dbl, "pulse_length":dbl, "detector":string, "Nchannels":i16, "ADCbits":i16, "BridgeVoltage (V)":sgl, "DAC Range Setting":u8, "AD 7730 Bit Settings":i32, "DAC and AD Settings":i32, "start time":i64, "Pre-start time (ms) of DAQ Typically set to 1000 ms":i32, "Measured Time for DAQ [ms] ":u32, "single channel number":i64, "maximum voltage @ 10MW single channel":dbl, "ExptSampleFrequency (Hz)":sgl, "single channel voltage factor":dbl, "CalibSampleFrequency (Hz)":sgl, "predicted time [ms] to finalize DAQ":dbl, "CalStep1 (V)":string, "CalStep2 (V)":string, "data string":string}[]
  T4 = cluster{"sample_period":dbl, "sample_rate":dbl, "pulse_length":dbl, "detector":string, "Nchannels":i16, "ADCbits":i16, "BridgeVoltage (V)":sgl, "DAC Range Setting":u8, "AD 7730 Bit Settings":i32, "DAC and AD Settings":i32, "start time":i64, "Pre-start time (ms) of DAQ Typically set to 1000 ms":i32, "Measured Time for DAQ [ms] ":u32, "single channel number":i64, "maximum voltage @ 10MW single channel":dbl, "ExptSampleFrequency (Hz)":sgl, "single channel voltage factor":dbl, "CalibSampleFrequency (Hz)":sgl, "predicted time [ms] to finalize DAQ":dbl, "CalStep1 (V)":string, "CalStep2 (V)":string, "data string":string}
  T5 = cluster{"name":string, "active":i32, "physicalQuantity":cluster{"type":string}}[]
  T6 = cluster{"chanDescs":cluster{"name":string, "active":i32}[]}[]
  T7 = cluster{"sample_period":dbl, "sample_rate":dbl, "pulse_length":dbl, "detector":string, "NChannels":i16, "ADCBits":i16, "BridgeVoltage (V)":sgl, "DAC Range Setting":u8, "AD 7730 Bit Settings":i32, "DAC and AD Settings":i32, "chanDescs":cluster{"name":string, "active":i32, "physicalQuantity":cluster{"type":string}}[], "start time":i64, "Pre-start time (ms) of DAQ Typically set to 1000 ms":i32, "Measured Time for DAQ [ms] ":u32, "single channel number":i64, "maximum voltage @ 10MW single channel":dbl, "ExptSampleFrequency (Hz)":sgl, "single channel voltage factor":dbl, "CalibSampleFrequency (Hz)":sgl, "predicted time [ms] to finalize DAQ":dbl, "CalStep1 (V)":string, "CalStep2 (V)":string, "data string":string}
  T8 = cluster{"sample_period":dbl, "sample_rate":dbl, "pulse_length":dbl, "detector":string, "NChannels":i16, "ADCBits":i16, "BridgeVoltage (V)":sgl, "DAC Range Setting":u8, "AD 7730 Bit Settings":i32, "DAC and AD Settings":i32, "start time":i64, "Pre-start time (ms) of DAQ Typically set to 1000 ms":i32, "Measured Time for DAQ [ms] ":u32, "single channel number":i64, "maximum voltage @ 10MW single channel":dbl, "ExptSampleFrequency (Hz)":sgl, "single channel voltage factor":dbl, "CalibSampleFrequency (Hz)":sgl, "predicted time [ms] to finalize DAQ":dbl, "CalStep1 (V)":string, "CalStep2 (V)":string, "data string":string}
  T9 = cluster{"sample_period":dbl, "sample_rate":dbl, "pulse_length":dbl, "detector":string, "NChannels":i16, "ADCBits":i16, "BridgeVoltage (V)":sgl, "DAC Range Setting":u8, "AD 7730 Bit Settings":i32, "DAC and AD Settings":i32, "start time":i64, "Pre-start time (ms) of DAQ Typically set to 1000 ms":i32, "Measured Time for DAQ [ms] ":u32, "single channel number":i64, "maximum voltage @ 10MW single channel":dbl, "ExptSampleFrequency (Hz)":sgl, "single channel voltage factor":dbl, "CalibSampleFrequency (Hz)":sgl, "predicted time [ms] to finalize DAQ":dbl, "CalStep1 (V)":string, "CalStep2 (V)":string, "data string":string}[]
  T10 = cluster{"sample_period":dbl, "sample_rate":dbl, "pulse_length":dbl, "detector":string, "NChannels":i16, "ADCBits":i16, "BridgeVoltage (V)":sgl, "DAC Range Setting":u8, "AD 7730 Bit Settings":i32, "DAC and AD Settings":i32, "chanDescs":cluster{"name":string, "active":i32, "physicalQuantity":cluster{"type":string}}[], "start time":i64, "Pre-start time (ms) of DAQ Typically set to 1000 ms":i32, "Measured Time for DAQ [ms] ":u32, "single channel number":i64, "maximum voltage @ 10MW single channel":dbl, "ExptSampleFrequency (Hz)":sgl, "single channel voltage factor":dbl, "CalibSampleFrequency (Hz)":sgl, "predicted time [ms] to finalize DAQ":dbl, "CalStep1 (V)":string, "CalStep2 (V)":string, "data string":string}[]
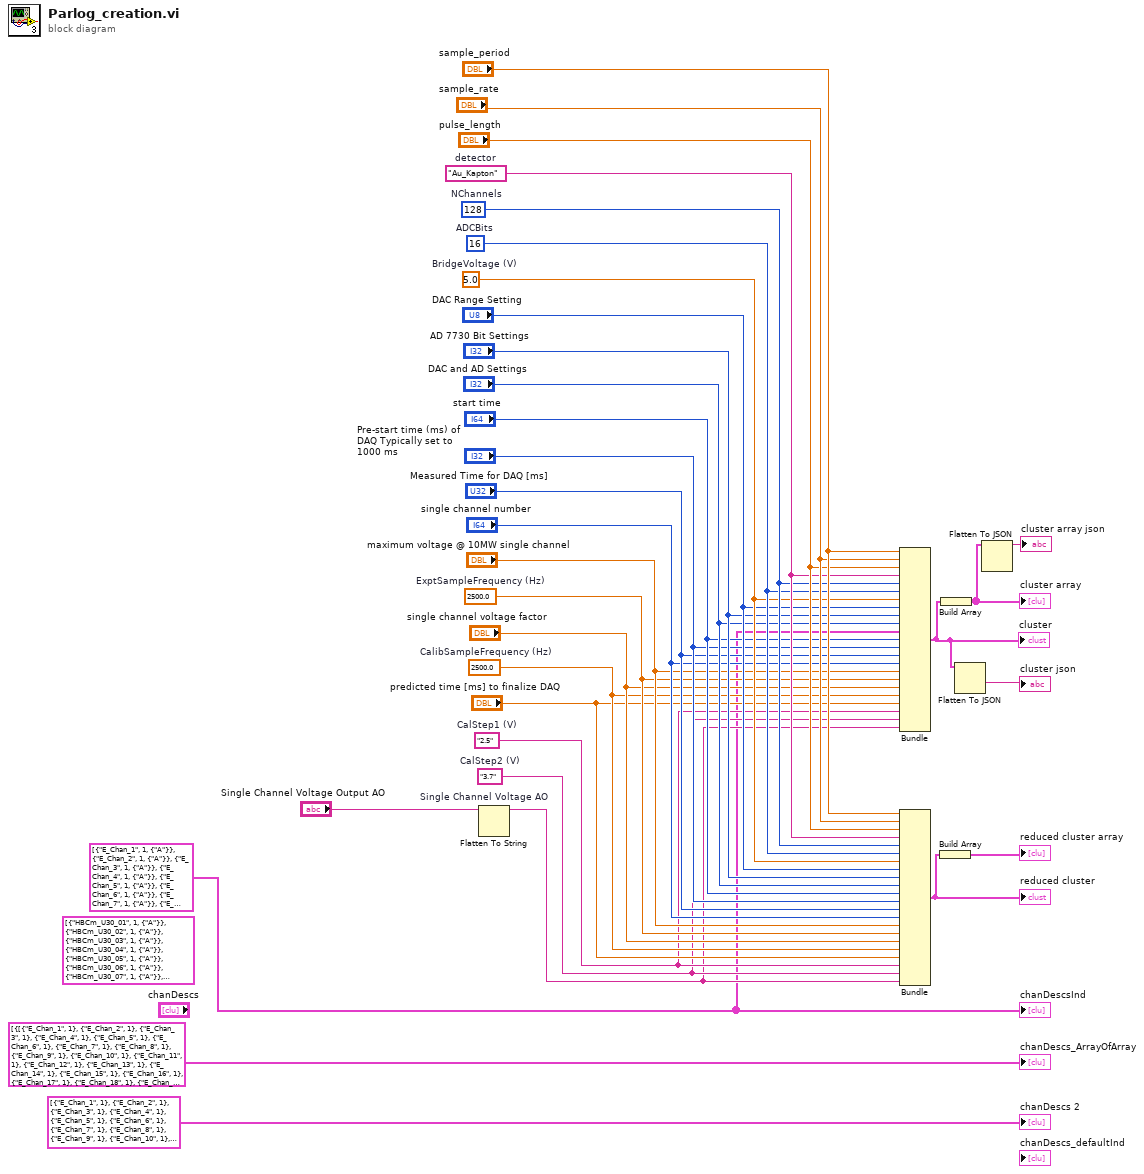
[diagram p0: block diagram]
diagram:
  w1 = T5 [{"name"="E_Chan_1", "active"=1, "physicalQuantity"={"type"="A"}}, {"name"="E_Chan_2", "active"=1, "physicalQuantity"={"type"="A"}}, {"name"="E_Chan_3", "active"=1, "physicalQuantity"={"type"="A"}}, {"name"="E_Chan_4", "active"=1, "physicalQuantity"={"type"="A"}}, {"name"="E_Chan_5", "active"=1, "physicalQuantity"={"type"="A"}}, {"name"="E_Chan_6", "active"=1, "physicalQuantity"={"type"="A"}}, {"name"="E_Chan_7", "active"=1, "physicalQuantity"={"type"="A"}}, {"name"="E_Chan_8", "active"=1, "physicalQuantity"={"type"="A"}}, {"name"="E_Chan_9", "active"=1, "physicalQuantity"={"type"="A"}}, {"name"="E_Chan_10", "active"=1, "physicalQuantity"={"type"="A"}}, {"name"="E_Chan_11", "active"=1, "physicalQuantity"={"type"="A"}}, {"name"="E_Chan_12", "active"=1, "physicalQuantity"={"type"="A"}}, {"name"="E_Chan_13", "active"=1, "physicalQuantity"={"type"="A"}}, {"name"="E_Chan_14", "active"=1, "physicalQuantity"={"type"="A"}}, {"name"="E_Chan_15", "active"=1, "physicalQuantity"={"type"="A"}}, {"name"="E_Chan_16", "active"=1, "physicalQuantity"={"type"="A"}}, {"name"="E_Chan_17", "active"=1, "physicalQuantity"={"type"="A"}}, {"name"="E_Chan_18", "active"=1, "physicalQuantity"={"type"="A"}}, {"name"="E_Chan_19", "active"=1, "physicalQuantity"={"type"="A"}}, {"name"="E_Chan_20", "active"=1, "physicalQuantity"={"type"="A"}}, {"name"="E_Chan_21", "active"=1, "physicalQuantity"={"type"="A"}}, {"name"="E_Chan_22", "active"=1, "physicalQuantity"={"type"="A"}}, {"name"="E_Chan_23", "active"=1, "physicalQuantity"={"type"="A"}}, {"name"="E_Chan_24", "active"=1, "physicalQuantity"={"type"="A"}}, {"name"="E_Chan_25", "active"=1, "physicalQuantity"={"type"="A"}}, {"name"="E_Chan_26", "active"=1, "physicalQuantity"={"type"="A"}}, {"name"="E_Chan_27", "active"=1, "physicalQuantity"={"type"="A"}}, {"name"="E_Chan_28", "active"=1, "physicalQuantity"={"type"="A"}}, {"name"="E_Chan_29", "active"=1, "physicalQuantity"={"type"="A"}}, {"name"="E_Chan_30", "active"=1, "physicalQuantity"={"type"="A"}}, {"name"="E_Chan_31", "active"=1, "physicalQuantity"={"type"="A"}}, {"name"="E_Chan_32", "active"=1, "physicalQuantity"={"type"="A"}}, {"name"="E_Chan_33", "active"=1, "physicalQuantity"={"type"="A"}}, {"name"="E_Chan_34", "active"=1, "physicalQuantity"={"type"="A"}}, {"name"="E_Chan_35", "active"=1, "physicalQuantity"={"type"="A"}}, {"name"="E_Chan_36", "active"=1, "physicalQuantity"={"type"="A"}}, {"name"="E_Chan_37", "active"=1, "physicalQuantity"={"type"="A"}}, {"name"="E_Chan_38", "active"=1, "physicalQuantity"={"type"="A"}}, {"name"="E_Chan_39", "active"=1, "physicalQuantity"={"type"="A"}}, {"name"="E_Chan_40", "active"=1, "physicalQuantity"={"type"="A"}}, {"name"="E_Chan_41", "active"=1, "physicalQuantity"={"type"="A"}}, {"name"="E_Chan_42", "active"=1, "physicalQuantity"={"type"="A"}}, {"name"="E_Chan_43", "active"=1, "physicalQuantity"={"type"="A"}}, {"name"="E_Chan_44", "active"=1, "physicalQuantity"={"type"="A"}}, {"name"="E_Chan_45", "active"=1, "physicalQuantity"={"type"="A"}}, {"name"="E_Chan_46", "active"=1, "physicalQuantity"={"type"="A"}}, {"name"="E_Chan_47", "active"=1, "physicalQuantity"={"type"="A"}}, {"name"="E_Chan_48", "active"=1, "physicalQuantity"={"type"="A"}}, {"name"="E_Chan_49", "active"=1, "physicalQuantity"={"type"="A"}}, {"name"="E_Chan_50", "active"=1, "physicalQuantity"={"type"="A"}}, {"name"="E_Chan_51", "active"=1, "physicalQuantity"={"type"="A"}}, {"name"="E_Chan_52", "active"=1, "physicalQuantity"={"type"="A"}}, {"name"="E_Chan_53", "active"=1, "physicalQuantity"={"type"="A"}}, {"name"="E_Chan_54", "active"=1, "physicalQuantity"={"type"="A"}}, {"name"="E_Chan_55", "active"=1, "physicalQuantity"={"type"="A"}}, {"name"="E_Chan_56", "active"=1, "physicalQuantity"={"type"="A"}}, {"name"="E_Chan_57", "active"=1, "physicalQuantity"={"type"="A"}}, {"name"="E_Chan_58", "active"=1, "physicalQuantity"={"type"="A"}}, {"name"="E_Chan_59", "active"=1, "physicalQuantity"={"type"="A"}}, {"name"="E_Chan_60", "active"=1, "physicalQuantity"={"type"="A"}}, {"name"="E_Chan_61", "active"=1, "physicalQuantity"={"type"="A"}}, {"name"="E_Chan_62", "active"=1, "physicalQuantity"={"type"="A"}}, {"name"="E_Chan_63", "active"=1, "physicalQuantity"={"type"="A"}}, {"name"="E_Chan_64", "active"=1, "physicalQuantity"={"type"="A"}}, {"name"="E_Chan_65", "active"=1, "physicalQuantity"={"type"="A"}}, {"name"="E_Chan_66", "active"=1, "physicalQuantity"={"type"="A"}}, {"name"="E_Chan_67", "active"=1, "physicalQuantity"={"type"="A"}}, {"name"="E_Chan_68", "active"=1, "physicalQuantity"={"type"="A"}}, {"name"="E_Chan_69", "active"=1, "physicalQuantity"={"type"="A"}}, {"name"="E_Chan_70", "active"=1, "physicalQuantity"={"type"="A"}}, {"name"="E_Chan_71", "active"=1, "physicalQuantity"={"type"="A"}}, {"name"="E_Chan_72", "active"=1, "physicalQuantity"={"type"="A"}}, {"name"="E_Chan_73", "active"=1, "physicalQuantity"={"type"="A"}}, {"name"="E_Chan_74", "active"=1, "physicalQuantity"={"type"="A"}}, {"name"="E_Chan_75", "active"=1, "physicalQuantity"={"type"="A"}}, {"name"="E_Chan_76", "active"=1, "physicalQuantity"={"type"="A"}}, {"name"="E_Chan_77", "active"=1, "physicalQuantity"={"type"="A"}}, {"name"="E_Chan_78", "active"=1, "physicalQuantity"={"type"="A"}}, {"name"="E_Chan_79", "active"=1, "physicalQuantity"={"type"="A"}}, {"name"="E_Chan_80", "active"=1, "physicalQuantity"={"type"="A"}}, {"name"="E_Chan_81", "active"=1, "physicalQuantity"={"type"="A"}}, {"name"="E_Chan_82", "active"=1, "physicalQuantity"={"type"="A"}}, {"name"="E_Chan_83", "active"=1, "physicalQuantity"={"type"="A"}}, {"name"="E_Chan_84", "active"=1, "physicalQuantity"={"type"="A"}}, {"name"="E_Chan_85", "active"=1, "physicalQuantity"={"type"="A"}}, {"name"="E_Chan_86", "active"=1, "physicalQuantity"={"type"="A"}}, {"name"="E_Chan_87", "active"=1, "physicalQuantity"={"type"="A"}}, {"name"="E_Chan_88", "active"=1, "physicalQuantity"={"type"="A"}}, {"name"="E_Chan_89", "active"=1, "physicalQuantity"={"type"="A"}}, {"name"="E_Chan_90", "active"=1, "physicalQuantity"={"type"="A"}}, {"name"="E_Chan_91", "active"=1, "physicalQuantity"={"type"="A"}}, {"name"="E_Chan_92", "active"=1, "physicalQuantity"={"type"="A"}}, {"name"="E_Chan_93", "active"=1, "physicalQuantity"={"type"="A"}}, {"name"="E_Chan_94", "active"=1, "physicalQuantity"={"type"="A"}}, {"name"="E_Chan_95", "active"=1, "physicalQuantity"={"type"="A"}}, {"name"="E_Chan_96", "active"=1, "physicalQuantity"={"type"="A"}}, {"name"="E_Chan_97", "active"=1, "physicalQuantity"={"type"="A"}}, {"name"="E_Chan_98", "active"=1, "physicalQuantity"={"type"="A"}}, {"name"="E_Chan_99", "active"=1, "physicalQuantity"={"type"="A"}}, {"name"="E_Chan_100", "active"=1, "physicalQuantity"={"type"="A"}}, {"name"="E_Chan_101", "active"=1, "physicalQuantity"={"type"="A"}}, {"name"="E_Chan_102", "active"=1, "physicalQuantity"={"type"="A"}}, {"name"="E_Chan_103", "active"=1, "physicalQuantity"={"type"="A"}}, {"name"="E_Chan_104", "active"=1, "physicalQuantity"={"type"="A"}}, {"name"="E_Chan_105", "active"=1, "physicalQuantity"={"type"="A"}}, {"name"="E_Chan_106", "active"=1, "physicalQuantity"={"type"="A"}}, {"name"="E_Chan_107", "active"=1, "physicalQuantity"={"type"="A"}}, {"name"="E_Chan_108", "active"=1, "physicalQuantity"={"type"="A"}}, {"name"="E_Chan_109", "active"=1, "physicalQuantity"={"type"="A"}}, {"name"="E_Chan_110", "active"=1, "physicalQuantity"={"type"="A"}}, {"name"="E_Chan_111", "active"=1, "physicalQuantity"={"type"="A"}}, {"name"="E_Chan_112", "active"=1, "physicalQuantity"={"type"="A"}}, {"name"="E_Chan_113", "active"=1, "physicalQuantity"={"type"="A"}}, {"name"="E_Chan_114", "active"=1, "physicalQuantity"={"type"="A"}}, {"name"="E_Chan_115", "active"=1, "physicalQuantity"={"type"="A"}}, {"name"="E_Chan_116", "active"=1, "physicalQuantity"={"type"="A"}}, {"name"="E_Chan_117", "active"=1, "physicalQuantity"={"type"="A"}}, {"name"="E_Chan_118", "active"=1, "physicalQuantity"={"type"="A"}}, {"name"="E_Chan_119", "active"=1, "physicalQuantity"={"type"="A"}}, {"name"="E_Chan_120", "active"=1, "physicalQuantity"={"type"="A"}}, {"name"="E_Chan_121", "active"=1, "physicalQuantity"={"type"="A"}}, {"name"="E_Chan_122", "active"=1, "physicalQuantity"={"type"="A"}}, {"name"="E_Chan_123", "active"=1, "physicalQuantity"={"type"="A"}}, {"name"="E_Chan_124", "active"=1, "physicalQuantity"={"type"="A"}}, {"name"="E_Chan_125", "active"=1, "physicalQuantity"={"type"="A"}}, {"name"="E_Chan_126", "active"=1, "physicalQuantity"={"type"="A"}}, {"name"="E_Chan_127", "active"=1, "physicalQuantity"={"type"="A"}}, {"name"="E_Chan_128", "active"=1, "physicalQuantity"={"type"="A"}}] ("chanDescs")
  (unwired) T5 [{"name"="HBCm_U30_01", "active"=1, "physicalQuantity"={"type"="A"}}, {"name"="HBCm_U30_02", "active"=1, "physicalQuantity"={"type"="A"}}, {"name"="HBCm_U30_03", "active"=1, "physicalQuantity"={"type"="A"}}, {"name"="HBCm_U30_04", "active"=1, "physicalQuantity"={"type"="A"}}, {"name"="HBCm_U30_05", "active"=1, "physicalQuantity"={"type"="A"}}, {"name"="HBCm_U30_06", "active"=1, "physicalQuantity"={"type"="A"}}, {"name"="HBCm_U30_07", "active"=1, "physicalQuantity"={"type"="A"}}, {"name"="HBCm_U30_08", "active"=1, "physicalQuantity"={"type"="A"}}, {"name"="HBCm_U30_09", "active"=1, "physicalQuantity"={"type"="A"}}, {"name"="HBCm_U30_10", "active"=1, "physicalQuantity"={"type"="A"}}, {"name"="HBCm_U30_11", "active"=1, "physicalQuantity"={"type"="A"}}, {"name"="HBCm_U30_12", "active"=1, "physicalQuantity"={"type"="A"}}, {"name"="HBCm_U30_013", "active"=1, "physicalQuantity"={"type"="A"}}, {"name"="HBCm_U30_14", "active"=1, "physicalQuantity"={"type"="A"}}, {"name"="HBCm_U30_15", "active"=1, "physicalQuantity"={"type"="A"}}, {"name"="HBCm_U30_16", "active"=1, "physicalQuantity"={"type"="A"}}, {"name"="HBCm_U30_17", "active"=1, "physicalQuantity"={"type"="A"}}, {"name"="HBCm_U30_18", "active"=1, "physicalQuantity"={"type"="A"}}, {"name"="HBCm_U30_19", "active"=1, "physicalQuantity"={"type"="A"}}, {"name"="HBCm_U30_20", "active"=1, "physicalQuantity"={"type"="A"}}, {"name"="HBCm_U30_21", "active"=1, "physicalQuantity"={"type"="A"}}, {"name"="HBCm_U30_22", "active"=1, "physicalQuantity"={"type"="A"}}, {"name"="HBCm_U30_23", "active"=1, "physicalQuantity"={"type"="A"}}, {"name"="HBCm_U30_24", "active"=1, "physicalQuantity"={"type"="A"}}, {"name"="HBCm_U30_25", "active"=1, "physicalQuantity"={"type"="A"}}, {"name"="HBCm_U30_26", "active"=1, "physicalQuantity"={"type"="A"}}, {"name"="HBCm_U30_27", "active"=1, "physicalQuantity"={"type"="A"}}, {"name"="HBCm_U30_28", "active"=1, "physicalQuantity"={"type"="A"}}, {"name"="HBCm_U30_29", "active"=1, "physicalQuantity"={"type"="A"}}, {"name"="HBCm_U30_30", "active"=1, "physicalQuantity"={"type"="A"}}, {"name"="HBCm_U30_31", "active"=1, "physicalQuantity"={"type"="A"}}, {"name"="HBCm_U30_32", "active"=1, "physicalQuantity"={"type"="A"}}, {"name"="VBCm_V21_01", "active"=1, "physicalQuantity"={"type"="A"}}, {"name"="VBCm_V21_02", "active"=1, "physicalQuantity"={"type"="A"}}, {"name"="VBCm_V21_03", "active"=1, "physicalQuantity"={"type"="A"}}, {"name"="VBCm_V21_04", "active"=1, "physicalQuantity"={"type"="A"}}, {"name"="VBCm_V21_05", "active"=1, "physicalQuantity"={"type"="A"}}, {"name"="VBCm_V21_06", "active"=1, "physicalQuantity"={"type"="A"}}, {"name"="VBCm_V21_07", "active"=1, "physicalQuantity"={"type"="A"}}, {"name"="VBCm_V21_08", "active"=1, "physicalQuantity"={"type"="A"}}, {"name"="VBCm_V21_09", "active"=1, "physicalQuantity"={"type"="A"}}, {"name"="VBCm_V21_10", "active"=1, "physicalQuantity"={"type"="A"}}, {"name"="VBCm_V21_11", "active"=1, "physicalQuantity"={"type"="A"}}, {"name"="VBCm_V21_12", "active"=1, "physicalQuantity"={"type"="A"}}, {"name"="VBCm_V21_13", "active"=1, "physicalQuantity"={"type"="A"}}, {"name"="VBCm_V21_14", "active"=1, "physicalQuantity"={"type"="A"}}, {"name"="VBCm_V21_15", "active"=1, "physicalQuantity"={"type"="A"}}, {"name"="VBCm_V21_16", "active"=1, "physicalQuantity"={"type"="A"}}, {"name"="VBCm_V21_17", "active"=1, "physicalQuantity"={"type"="A"}}, {"name"="VBCm_V21_18", "active"=1, "physicalQuantity"={"type"="A"}}, {"name"="VBCm_V21_19", "active"=1, "physicalQuantity"={"type"="A"}}, {"name"="VBCm_V21_20", "active"=1, "physicalQuantity"={"type"="A"}}, {"name"="VBCm_V21_21", "active"=1, "physicalQuantity"={"type"="A"}}, {"name"="VBCm_V21_22", "active"=1, "physicalQuantity"={"type"="A"}}, {"name"="VBCm_V21_23", "active"=1, "physicalQuantity"={"type"="A"}}, {"name"="VBCm_V21_24", "active"=1, "physicalQuantity"={"type"="A"}}, {"name"="VBCm_V21_25", "active"=1, "physicalQuantity"={"type"="A"}}, {"name"="VBCm_V21_26", "active"=1, "physicalQuantity"={"type"="A"}}, {"name"="VBCm_V21_27", "active"=1, "physicalQuantity"={"type"="A"}}, {"name"="VBCm_V21_28", "active"=1, "physicalQuantity"={"type"="A"}}, {"name"="VBCm_V21_29", "active"=1, "physicalQuantity"={"type"="A"}}, {"name"="VBCm_V21_30", "active"=1, "physicalQuantity"={"type"="A"}}, {"name"="VBCm_V21_31", "active"=1, "physicalQuantity"={"type"="A"}}, {"name"="VBCm_V21_32", "active"=1, "physicalQuantity"={"type"="A"}}, {"name"="VBCm_V21_33", "active"=1, "physicalQuantity"={"type"="A"}}, {"name"="VBCm_V21_34", "active"=1, "physicalQuantity"={"type"="A"}}, {"name"="VBCm_V21_35", "active"=1, "physicalQuantity"={"type"="A"}}, {"name"="VBCm_V21_36", "active"=1, "physicalQuantity"={"type"="A"}}, {"name"="VBCm_V21_37", "active"=1, "physicalQuantity"={"type"="A"}}, {"name"="VBCm_V21_38", "active"=1, "physicalQuantity"={"type"="A"}}, {"name"="VBCm_V21_39", "active"=1, "physicalQuantity"={"type"="A"}}, {"name"="VBCm_V21_40", "active"=1, "physicalQuantity"={"type"="A"}}, {"name"="VBCs_V21_01", "active"=1, "physicalQuantity"={"type"="A"}}, {"name"="VBCs_V21_02", "active"=1, "physicalQuantity"={"type"="A"}}, {"name"="VBCs_V21_03", "active"=1, "physicalQuantity"={"type"="A"}}, {"name"="VBCs_V21_04", "active"=1, "physicalQuantity"={"type"="A"}}, {"name"="VBCs_V21_05", "active"=1, "physicalQuantity"={"type"="A"}}, {"name"="VBCs_V21_06", "active"=1, "physicalQuantity"={"type"="A"}}, {"name"="VBCs_V21_07", "active"=1, "physicalQuantity"={"type"="A"}}, {"name"="VBCs_V21_08", "active"=1, "physicalQuantity"={"type"="A"}}, {"name"="HBCs_U30_01", "active"=1, "physicalQuantity"={"type"="A"}}, {"name"="HBCs_U30_02", "active"=1, "physicalQuantity"={"type"="A"}}, {"name"="HBCs_U30_03", "active"=1, "physicalQuantity"={"type"="A"}}, {"name"="HBCs_U30_04", "active"=1, "physicalQuantity"={"type"="A"}}, {"name"="HBCs_U30_05", "active"=1, "physicalQuantity"={"type"="A"}}, {"name"="HBCs_U30_06", "active"=1, "physicalQuantity"={"type"="A"}}, {"name"="HBCs_U30_07", "active"=1, "physicalQuantity"={"type"="A"}}, {"name"="HBCs_U30_08", "active"=1, "physicalQuantity"={"type"="A"}}, {"name"="HBCs_U30_09", "active"=1, "physicalQuantity"={"type"="A"}}, {"name"="HBCs_U30_10", "active"=1, "physicalQuantity"={"type"="A"}}, {"name"="HBCs_U30_11", "active"=1, "physicalQuantity"={"type"="A"}}, {"name"="HBCs_U30_12", "active"=1, "physicalQuantity"={"type"="A"}}, {"name"="HBCs_U30_13", "active"=1, "physicalQuantity"={"type"="A"}}, {"name"="HBCs_U30_14", "active"=1, "physicalQuantity"={"type"="A"}}, {"name"="HBCs_U30_15", "active"=1, "physicalQuantity"={"type"="A"}}, {"name"="HBCs_U30_16", "active"=1, "physicalQuantity"={"type"="A"}}] ("chanDescs")
  w28 = "Au_Kapton"  # detector
  w11 = "3.7"  # CalStep2 (V)
  w12 = "2.5"  # CalStep1 (V)
  w14 = sgl 2500.0  # CalibSampleFrequency (Hz)
  w16 = sgl 2500.0  # ExptSampleFrequency (Hz)
  w25 = sgl 5.0  # BridgeVoltage (V)
  w26 = i16 16  # ADCBits
  w27 = i16 128  # NChannels
  n1 = Flatten To String "Single Channel Voltage AO"(anything="Single Channel Voltage Output AO") -> (data string=w10:string)  [unwired: 3 in, 2 out]
  n2 = Bundle("sample_period"="sample_period", "sample_rate"="sample_rate", "pulse_length"="pulse_length", "detector"=w28, "NChannels"=w27, "ADCBits"=w26, "BridgeVoltage (V)"=w25, "DAC Range Setting"="DAC Range Setting", "AD 7730 Bit Settings"="AD 7730 Bit Settings", "DAC and AD Settings"="DAC and AD Settings", "chanDescs"=w1, "start time"="start time", "Pre-start time (ms) of DAQ Typically set to 1000 ms"="Pre-start time (ms) of DAQ Typically set to 1000 ms", "Measured Time for DAQ [ms]"="Measured Time for DAQ [ms]", "single channel number"="single channel number", "maximum voltage @ 10MW single channel"="maximum voltage @ 10MW single channel", "ExptSampleFrequency (Hz)"=w16, "single channel voltage factor"="single channel voltage factor", "CalibSampleFrequency (Hz)"=w14, "predicted time [ms] to finalize DAQ"="predicted time [ms] to finalize DAQ", "CalStep1 (V)"=w12, "CalStep2 (V)"=w11, "data string"=w10) -> (w3:T7)  [unwired: 1 in]
  "cluster" <- w3
  n3 = Bundle("sample_period"="sample_period", "sample_rate"="sample_rate", "pulse_length"="pulse_length", "detector"=w28, "NChannels"=w27, "ADCBits"=w26, "BridgeVoltage (V)"=w25, "DAC Range Setting"="DAC Range Setting", "AD 7730 Bit Settings"="AD 7730 Bit Settings", "DAC and AD Settings"="DAC and AD Settings", "start time"="start time", "Pre-start time (ms) of DAQ Typically set to 1000 ms"="Pre-start time (ms) of DAQ Typically set to 1000 ms", "Measured Time for DAQ [ms]"="Measured Time for DAQ [ms]", "single channel number"="single channel number", "maximum voltage @ 10MW single channel"="maximum voltage @ 10MW single channel", "ExptSampleFrequency (Hz)"=w16, "single channel voltage factor"="single channel voltage factor", "CalibSampleFrequency (Hz)"=w14, "predicted time [ms] to finalize DAQ"="predicted time [ms] to finalize DAQ", "CalStep1 (V)"=w12, "CalStep2 (V)"=w11, "data string"=w10) -> (w9:T8)  [unwired: 1 in]
  "reduced cluster" <- w9
  n4 = Build Array(w9) -> (→"reduced cluster array":T9)
  n5 = Build Array(w3) -> (w5:T10)
  "cluster array" <- w5
  n6 = Flatten To JSON(anything=w3) -> (JSON string=→"cluster json":string)  [unwired: 2 in, 1 out]
  n7 = Flatten To JSON(anything=w5) -> (JSON string=→"cluster array json":string)  [unwired: 2 in, 1 out]
  "chanDescs_ArrayOfArray" <- T6 [{"chanDescs"=[{"name"="E_Chan_1", "active"=1}, {"name"="E_Chan_2", "active"=1}, {"name"="E_Chan_3", "active"=1}, {"name"="E_Chan_4", "active"=1}, {"name"="E_Chan_5", "active"=1}, {"name"="E_Chan_6", "active"=1}, {"name"="E_Chan_7", "active"=1}, {"name"="E_Chan_8", "active"=1}, {"name"="E_Chan_9", "active"=1}, {"name"="E_Chan_10", "active"=1}, {"name"="E_Chan_11", "active"=1}, {"name"="E_Chan_12", "active"=1}, {"name"="E_Chan_13", "active"=1}, {"name"="E_Chan_14", "active"=1}, {"name"="E_Chan_15", "active"=1}, {"name"="E_Chan_16", "active"=1}, {"name"="E_Chan_17", "active"=1}, {"name"="E_Chan_18", "active"=1}, {"name"="E_Chan_19", "active"=1}, {"name"="E_Chan_20", "active"=1}, {"name"="E_Chan_21", "active"=1}, {"name"="E_Chan_22", "active"=1}, {"name"="E_Chan_23", "active"=1}, {"name"="E_Chan_24", "active"=1}, {"name"="E_Chan_25", "active"=1}, {"name"="E_Chan_26", "active"=1}, {"name"="E_Chan_27", "active"=1}, {"name"="E_Chan_28", "active"=1}, {"name"="E_Chan_29", "active"=1}, {"name"="E_Chan_30", "active"=1}, {"name"="E_Chan_31", "active"=1}, {"name"="E_Chan_32", "active"=1}, {"name"="E_Chan_33", "active"=1}, {"name"="E_Chan_34", "active"=1}, {"name"="E_Chan_35", "active"=1}, {"name"="E_Chan_36", "active"=1}, {"name"="E_Chan_37", "active"=1}, {"name"="E_Chan_38", "active"=1}, {"name"="E_Chan_39", "active"=1}, {"name"="E_Chan_40", "active"=1}, {"name"="E_Chan_41", "active"=1}, {"name"="E_Chan_42", "active"=1}, {"name"="E_Chan_43", "active"=1}, {"name"="E_Chan_44", "active"=1}, {"name"="E_Chan_45", "active"=1}, {"name"="E_Chan_46", "active"=1}, {"name"="E_Chan_47", "active"=1}, {"name"="E_Chan_48", "active"=1}, {"name"="E_Chan_49", "active"=1}, {"name"="E_Chan_50", "active"=1}, {"name"="E_Chan_51", "active"=1}, {"name"="E_Chan_52", "active"=1}, {"name"="E_Chan_53", "active"=1}, {"name"="E_Chan_54", "active"=1}, {"name"="E_Chan_55", "active"=1}, {"name"="E_Chan_56", "active"=1}, {"name"="E_Chan_57", "active"=1}, {"name"="E_Chan_58", "active"=1}, {"name"="E_Chan_59", "active"=1}, {"name"="E_Chan_60", "active"=1}, {"name"="E_Chan_61", "active"=1}, {"name"="E_Chan_62", "active"=1}, {"name"="E_Chan_63", "active"=1}, {"name"="E_Chan_64", "active"=1}, {"name"="E_Chan_65", "active"=1}, {"name"="E_Chan_66", "active"=1}, {"name"="E_Chan_67", "active"=1}, {"name"="E_Chan_68", "active"=1}, {"name"="E_Chan_69", "active"=1}, {"name"="E_Chan_70", "active"=1}, {"name"="E_Chan_71", "active"=1}, {"name"="E_Chan_72", "active"=1}, {"name"="E_Chan_73", "active"=1}, {"name"="E_Chan_74", "active"=1}, {"name"="E_Chan_75", "active"=1}, {"name"="E_Chan_76", "active"=1}, {"name"="E_Chan_77", "active"=1}, {"name"="E_Chan_78", "active"=1}, {"name"="E_Chan_79", "active"=1}, {"name"="E_Chan_80", "active"=1}, {"name"="E_Chan_81", "active"=1}, {"name"="E_Chan_82", "active"=1}, {"name"="E_Chan_83", "active"=1}, {"name"="E_Chan_84", "active"=1}, {"name"="E_Chan_85", "active"=1}, {"name"="E_Chan_86", "active"=1}, {"name"="E_Chan_87", "active"=1}, {"name"="E_Chan_88", "active"=1}, {"name"="E_Chan_89", "active"=1}, {"name"="E_Chan_90", "active"=1}, {"name"="E_Chan_91", "active"=1}, {"name"="E_Chan_92", "active"=1}, {"name"="E_Chan_93", "active"=1}, {"name"="E_Chan_94", "active"=1}, {"name"="E_Chan_95", "active"=1}, {"name"="E_Chan_96", "active"=1}, {"name"="E_Chan_97", "active"=1}, {"name"="E_Chan_98", "active"=1}, {"name"="E_Chan_99", "active"=1}, {"name"="E_Chan_100", "active"=1}, {"name"="E_Chan_101", "active"=1}, {"name"="E_Chan_102", "active"=1}, {"name"="E_Chan_103", "active"=1}, {"name"="E_Chan_104", "active"=1}, {"name"="E_Chan_105", "active"=1}, {"name"="E_Chan_106", "active"=1}, {"name"="E_Chan_107", "active"=1}, {"name"="E_Chan_108", "active"=1}, {"name"="E_Chan_109", "active"=1}, {"name"="E_Chan_110", "active"=1}, {"name"="E_Chan_111", "active"=1}, {"name"="E_Chan_112", "active"=1}, {"name"="E_Chan_113", "active"=1}, {"name"="E_Chan_114", "active"=1}, {"name"="E_Chan_115", "active"=1}, {"name"="E_Chan_116", "active"=1}, {"name"="E_Chan_117", "active"=1}, {"name"="E_Chan_118", "active"=1}, {"name"="E_Chan_119", "active"=1}, {"name"="E_Chan_120", "active"=1}, {"name"="E_Chan_121", "active"=1}, {"name"="E_Chan_122", "active"=1}, {"name"="E_Chan_123", "active"=1}, {"name"="E_Chan_124", "active"=1}, {"name"="E_Chan_125", "active"=1}, {"name"="E_Chan_126", "active"=1}, {"name"="E_Chan_127", "active"=1}, {"name"="E_Chan_128", "active"=1}]}] ("values")
  "chanDescsInd" <- w1
  "chanDescs 2" <- cluster{"name":string, "active":i32}[] [{"name"="E_Chan_1", "active"=1}, {"name"="E_Chan_2", "active"=1}, {"name"="E_Chan_3", "active"=1}, {"name"="E_Chan_4", "active"=1}, {"name"="E_Chan_5", "active"=1}, {"name"="E_Chan_6", "active"=1}, {"name"="E_Chan_7", "active"=1}, {"name"="E_Chan_8", "active"=1}, {"name"="E_Chan_9", "active"=1}, {"name"="E_Chan_10", "active"=1}, {"name"="E_Chan_11", "active"=1}, {"name"="E_Chan_12", "active"=1}, {"name"="E_Chan_13", "active"=1}, {"name"="E_Chan_14", "active"=1}, {"name"="E_Chan_15", "active"=1}, {"name"="E_Chan_16", "active"=1}, {"name"="E_Chan_17", "active"=1}, {"name"="E_Chan_18", "active"=1}, {"name"="E_Chan_19", "active"=1}, {"name"="E_Chan_20", "active"=1}, {"name"="E_Chan_21", "active"=1}, {"name"="E_Chan_22", "active"=1}, {"name"="E_Chan_23", "active"=1}, {"name"="E_Chan_24", "active"=1}, {"name"="E_Chan_25", "active"=1}, {"name"="E_Chan_26", "active"=1}, {"name"="E_Chan_27", "active"=1}, {"name"="E_Chan_28", "active"=1}, {"name"="E_Chan_29", "active"=1}, {"name"="E_Chan_30", "active"=1}, {"name"="E_Chan_31", "active"=1}, {"name"="E_Chan_32", "active"=1}, {"name"="E_Chan_33", "active"=1}, {"name"="E_Chan_34", "active"=1}, {"name"="E_Chan_35", "active"=1}, {"name"="E_Chan_36", "active"=1}, {"name"="E_Chan_37", "active"=1}, {"name"="E_Chan_38", "active"=1}, {"name"="E_Chan_39", "active"=1}, {"name"="E_Chan_40", "active"=1}, {"name"="E_Chan_41", "active"=1}, {"name"="E_Chan_42", "active"=1}, {"name"="E_Chan_43", "active"=1}, {"name"="E_Chan_44", "active"=1}, {"name"="E_Chan_45", "active"=1}, {"name"="E_Chan_46", "active"=1}, {"name"="E_Chan_47", "active"=1}, {"name"="E_Chan_48", "active"=1}, {"name"="E_Chan_49", "active"=1}, {"name"="E_Chan_50", "active"=1}, {"name"="E_Chan_51", "active"=1}, {"name"="E_Chan_52", "active"=1}, {"name"="E_Chan_53", "active"=1}, {"name"="E_Chan_54", "active"=1}, {"name"="E_Chan_55", "active"=1}, {"name"="E_Chan_56", "active"=1}, {"name"="E_Chan_57", "active"=1}, {"name"="E_Chan_58", "active"=1}, {"name"="E_Chan_59", "active"=1}, {"name"="E_Chan_60", "active"=1}, {"name"="E_Chan_61", "active"=1}, {"name"="E_Chan_62", "active"=1}, {"name"="E_Chan_63", "active"=1}, {"name"="E_Chan_64", "active"=1}, {"name"="E_Chan_65", "active"=1}, {"name"="E_Chan_66", "active"=1}, {"name"="E_Chan_67", "active"=1}, {"name"="E_Chan_68", "active"=1}, {"name"="E_Chan_69", "active"=1}, {"name"="E_Chan_70", "active"=1}, {"name"="E_Chan_71", "active"=1}, {"name"="E_Chan_72", "active"=1}, {"name"="E_Chan_73", "active"=1}, {"name"="E_Chan_74", "active"=1}, {"name"="E_Chan_75", "active"=1}, {"name"="E_Chan_76", "active"=1}, {"name"="E_Chan_77", "active"=1}, {"name"="E_Chan_78", "active"=1}, {"name"="E_Chan_79", "active"=1}, {"name"="E_Chan_80", "active"=1}, {"name"="E_Chan_81", "active"=1}, {"name"="E_Chan_82", "active"=1}, {"name"="E_Chan_83", "active"=1}, {"name"="E_Chan_84", "active"=1}, {"name"="E_Chan_85", "active"=1}, {"name"="E_Chan_86", "active"=1}, {"name"="E_Chan_87", "active"=1}, {"name"="E_Chan_88", "active"=1}, {"name"="E_Chan_89", "active"=1}, {"name"="E_Chan_90", "active"=1}, {"name"="E_Chan_91", "active"=1}, {"name"="E_Chan_92", "active"=1}, {"name"="E_Chan_93", "active"=1}, {"name"="E_Chan_94", "active"=1}, {"name"="E_Chan_95", "active"=1}, {"name"="E_Chan_96", "active"=1}, {"name"="E_Chan_97", "active"=1}, {"name"="E_Chan_98", "active"=1}, {"name"="E_Chan_99", "active"=1}, {"name"="E_Chan_100", "active"=1}, {"name"="E_Chan_101", "active"=1}, {"name"="E_Chan_102", "active"=1}, {"name"="E_Chan_103", "active"=1}, {"name"="E_Chan_104", "active"=1}, {"name"="E_Chan_105", "active"=1}, {"name"="E_Chan_106", "active"=1}, {"name"="E_Chan_107", "active"=1}, {"name"="E_Chan_108", "active"=1}, {"name"="E_Chan_109", "active"=1}, {"name"="E_Chan_110", "active"=1}, {"name"="E_Chan_111", "active"=1}, {"name"="E_Chan_112", "active"=1}, {"name"="E_Chan_113", "active"=1}, {"name"="E_Chan_114", "active"=1}, {"name"="E_Chan_115", "active"=1}, {"name"="E_Chan_116", "active"=1}, {"name"="E_Chan_117", "active"=1}, {"name"="E_Chan_118", "active"=1}, {"name"="E_Chan_119", "active"=1}, {"name"="E_Chan_120", "active"=1}, {"name"="E_Chan_121", "active"=1}, {"name"="E_Chan_122", "active"=1}, {"name"="E_Chan_123", "active"=1}, {"name"="E_Chan_124", "active"=1}, {"name"="E_Chan_125", "active"=1}, {"name"="E_Chan_126", "active"=1}, {"name"="E_Chan_127", "active"=1}, {"name"="E_Chan_128", "active"=1}] ("chanDescs")
